vi "MSTR_Bool_To_String.vi"(11 "Boolean in":bool) -> (3 "String Boolean out":string)   [LabVIEW 2018]
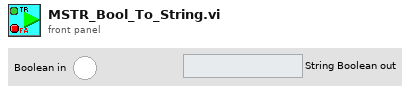
[diagram p1: front panel]
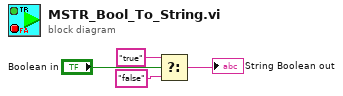
[diagram p0: block diagram]
diagram:
  n1 = Select(t="true", s="Boolean in", f="false") -> (s? t:f=→"String Boolean out":string)
